vi "PULSE_OXIMETER.vi"() -> ()   [LabVIEW 2013]
uses:
  <vilib>/Instr/_visa.llb/VISA Configure Serial Port (Instr).vi
panel:
  out "Inicial Time":u32
  out "Valor Medio":string
  out "SpO2":string
  in  "A":dbl=110.0 format="%#_13g"
  in  "B":dbl=25.0 format="%#_13g"
  out "Light Intensity RED 2":i64(slide) scale=0.0..100.0
  in  "Light Intensity RED":i16(slide) scale=0.0..100.0
  out "RED":i32(graph)
  out "Light Intensity IR 2":i64(slide) scale=0.0..100.0
  out "JSON string 2":string
  out "error out":errorcluster
  out "IR":i32(graph)
  out "JSON string":string
  in  "Light Intensity IR":i64(slide) scale=0.0..100.0
  in  "Light Intensity Mode":bool
  out "AMB":i32
  out "IR":i32
  out "RED":i32
  in  "Read Count":u32=1000
  in  "End Write on Termination Character?":bool=TRUE
  in  "End Read on Termination Character?":bool=TRUE
  in  "Termination Character":u8=10 format="%.0x"
  in  "PUERTO":refnum<visa-resource-name>
  in  "START/STOP":bool
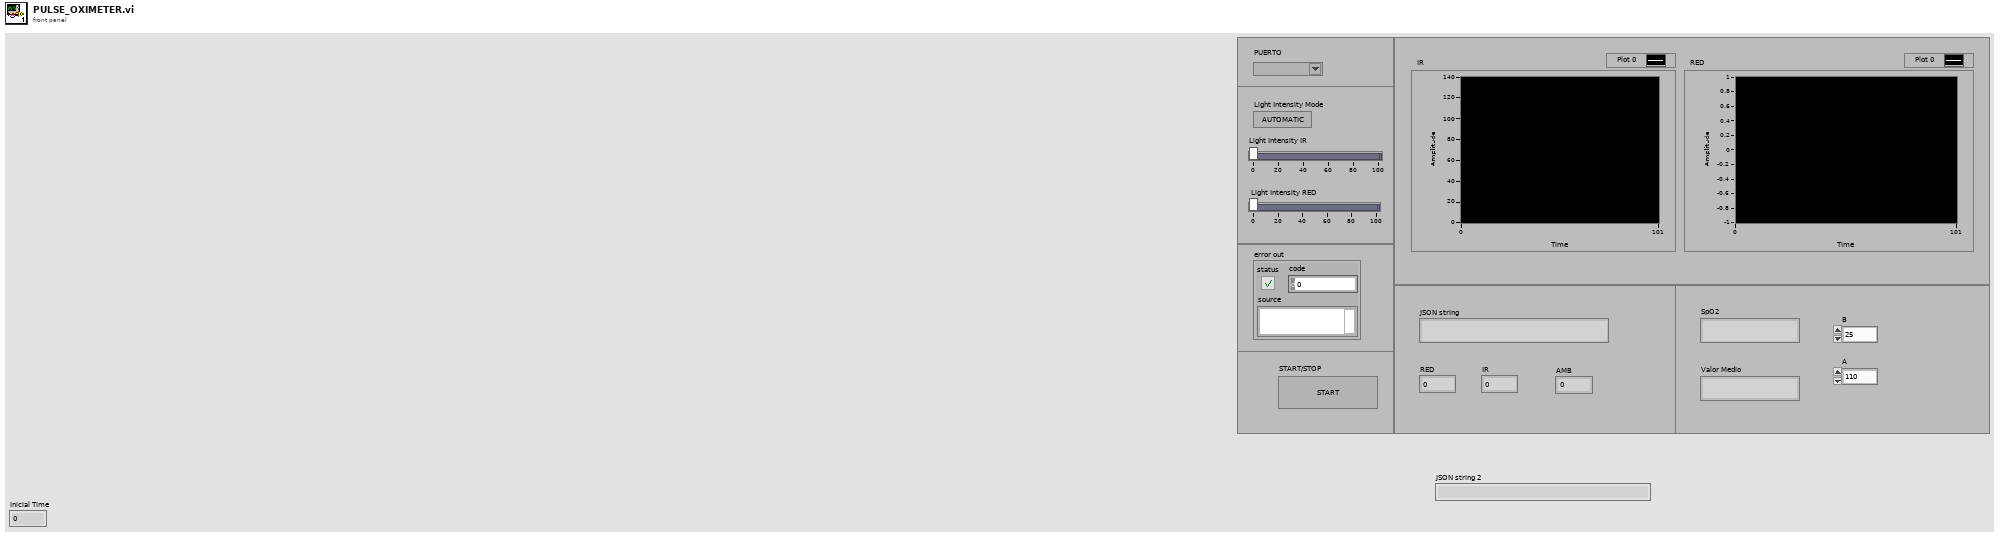
[diagram p1: front panel]
types:
  T1 = cluster{"mode":bool, "LightIntensity_IR":dbl, "status":bool, "LightIntensity_RED":dbl}
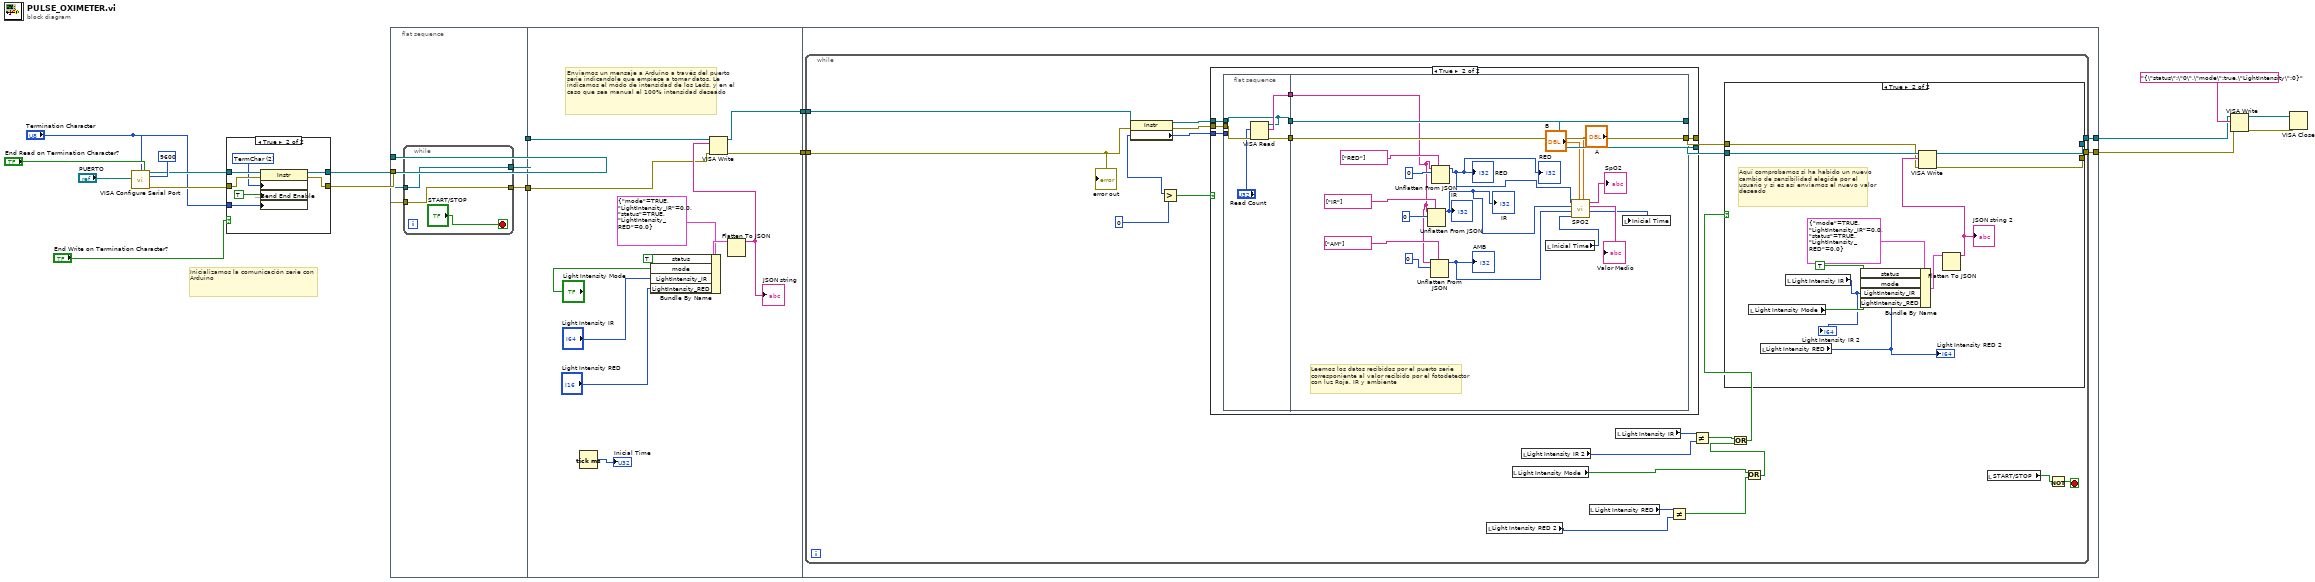
[diagram p0: block diagram]
diagram:
  # "Inicializamos la comunicación serie con Arduino"
  n1 = call-poly "VISA Configure Serial Port"("VISA resource name"="PUERTO", "termination char\n(0xA = '\\n' = LF)"="Termination Character", "Enable Termination\nChar (T)"="End Read on Termination Character?", "baud rate (9600)"=u32 9600) -> ("VISA resource name out"=w13:refnum<visa-resource-name>, "error out"=w12:errorcluster)  [unwired: 10 in]
  n2 = case shown="True" "End Write on Termination Character?" {
    tunnel: w13 -> [w19 w27]
    tunnel: w12 -> [w20 w26]
    tunnel: [w19 w25] -> w15
    tunnel: [w20 w24] -> w14
    tunnel: "Termination Character" -> [_ w22]
    frame False {
    }
    frame True {
      w23 = u16 2 items=["None", "LastBit", "TermChar", "Break"] ("Serial Settings:Serial End Mode for Writes")
      n3 = property class="Instr"(reference=w27, error in=w26, "Serial Settings:End Mode for Writes"=w23, "Message Based Settings:Send End Enable"=TRUE, "Message Based Settings:Termination Character"=w22) -> (reference out=w25:refnum<visa-resource-name>, error out=w24:errorcluster)
    }
  }
  n4 = flat-sequence {
    tunnel: w15 -> [w31]
    tunnel: w14 -> [w30]
    tunnel: [w29] -> w6
    tunnel: [w28] -> w4
    tunnel: w6 -> [w41]
    tunnel: [w40] -> w5
    tunnel: w4 -> [w39]
    tunnel: [w38] -> w3
    tunnel: w5 -> [w50]
    tunnel: w3 -> [w49]
    tunnel: [w48] -> w2
    tunnel: [w47] -> w1
    frame #0 {
      n5 = while {
        tunnel: [w34] -> w29
        tunnel: w31 -> [w34]
        tunnel: [w33] -> w28
        tunnel: w30 -> [w33]
        stop <- "START/STOP" stop-if-true
      }
    }
    frame #1 {
      # "Enviamos un mensaje a Arduino a través del puerto serie indicandole que empiece a tomar datos. Le indicamos el módo de intensidad de los Leds, y en el caso que sea manual el 100% intensidad deseado"
      n6 = Tick Count (ms)() -> (millisecond timer value=→"Inicial Time":u32)
      n7 = Bundle By Name(cluster=T1 {"mode"=TRUE, "LightIntensity_IR"=0.0, "status"=TRUE, "LightIntensity_RED"=0.0} ("input cluster"), "status"=TRUE, "mode"="Light Intensity Mode", "LightIntensity_IR"="Light Intensity IR", "LightIntensity_RED"="Light Intensity RED") -> (w46:T1)
      n8 = Flatten To JSON(anything=w46) -> (JSON string=w44:string)  [unwired: 2 in, 1 out]
      "JSON string" <- w44
      n9 = VISA Write(VISA resource name=w41, write buffer=w44, error in (no error)=w39) -> (VISA resource name out=w40:refnum<visa-resource-name>, error out=w38:errorcluster)  [unwired: 1 out]
    }
    frame #2 {
      n10 = while {
        tunnel: w50 -> [w68]
        tunnel: w49 -> [w67]
        tunnel: [w65] -> w48
        tunnel: [w64] -> w47
        stop <- w70 stop-if-true
        n11 = property class="Instr"(reference=w68, error in=w67) -> (reference out=w69:refnum<visa-resource-name>, error out=w72:errorcluster, "Serial Settings:Number of Bytes at Serial Port"=w59:u32)
        n12 = Greater?(x=w59, y=u32 0) -> (0:w60:bool)
        n13 = case shown="True" w60 {
          tunnel: w72 -> [w73 w79]
          tunnel: w59 -> [_ w78]
          tunnel: w69 -> [w74 w77]
          tunnel: [w74 w76] -> w66
          tunnel: [w73 w75] -> w63
          frame False {
          }
          frame True {
            n14 = flat-sequence {
              tunnel: w79 -> [w87]
              tunnel: w78 -> [_]
              tunnel: w77 -> [w84]
              tunnel: [w86] -> w82
              tunnel: [w85] -> w81
              tunnel: [w84] -> w80
              tunnel: [w105] -> w75
              tunnel: w82 -> [w97]
              tunnel: w81 -> [w105]
              tunnel: [w104] -> w76
              tunnel: w80 -> [w104]
              frame #0 {
                n15 = VISA Read(VISA resource name=w84, byte count="Read Count", error in (no error)=w87) -> (read buffer=w86:string, error out=w85:errorcluster)  [unwired: 2 out]
              }
              frame #1 {
                # "Leemos los datos recibidos por el puerto serie corresponiente al valor recibido por el fotodetector con luz Roja, IR y ambiente"
                n16 = Unflatten From JSON(path=string[] ["IR"] ("path 2"), JSON string=w97, type and defaults=0) -> (value=w95:i32)  [unwired: 4 in, 1 out]
                "IR" <- w95
                "IR" <- w95
                n17 = Unflatten From JSON(path=string[] ["AM"] ("path 2"), JSON string=w97, type and defaults=0) -> (value=w94:i32)  [unwired: 4 in, 1 out]
                "AMB" <- w94
                n18 = Unflatten From JSON(path=string[] ["RED"] ("path 2"), JSON string=w97, type and defaults=0) -> (value=w96:i32)  [unwired: 4 in, 1 out]
                "RED" <- w96
                "RED" <- w96
                n19 = local read "Inicial Time"() -> (w89:u32)
                n20 = call "SPO2.vi"("A"="A", "B"="B", "Inicial"=w89, "AMB"=w94, "IR"=w95, "RED"=w96) -> ("Inicial Time Out"=w88:u32, "Valor Medio"=→"Valor Medio":string, "SpO2"=→"SpO2":string)  [unwired: 3 in]
                n21 = local write "Inicial Time"(w88) -> ()
              }
            }
          }
        }
        n22 = local read "Light Intensity RED 2"() -> (w55:i64)
        n23 = local read "Light Intensity Mode"() -> (w52:bool)
        n24 = local read "Light Intensity IR 2"() -> (w61:i64)
        n25 = local read "Light Intensity RED"() -> (w56:i16)
        n26 = local read "Light Intensity IR"() -> (w62:i64)
        n27 = Not Equal?(x=w56, y=w55) -> (x != y?=w54:bool)
        n28 = Not Equal?(x=w62, y=w61) -> (x != y?=w57:bool)
        n29 = Or(x=w52, y=w54) -> (x .or. y?=w51:bool)
        n30 = Or(x=w57, y=w51) -> (x .or. y?=w53:bool)
        n31 = case shown="True" w53 {
          tunnel: w66 -> [w106 w116]
          tunnel: [w106 w115] -> w65
          tunnel: [w107 w114] -> w64
          tunnel: w63 -> [w107 w113]
          frame False {
          }
          frame True {
            # "Aquí comprobamos si ha habido un nuevo cambio de sensibilidad elegida por el usuario y si es así enviamos el nuevo valor deseado"
            n32 = local read "Light Intensity Mode"() -> (w112:bool)
            n33 = local read "Light Intensity RED"() -> (w108:i16)
            "Light Intensity RED 2" <- w108
            n34 = local read "Light Intensity IR"() -> (w111:i64)
            "Light Intensity IR 2" <- w111
            n35 = Bundle By Name(cluster=T1 {"mode"=TRUE, "LightIntensity_IR"=0.0, "status"=TRUE, "LightIntensity_RED"=0.0} ("input cluster"), "status"=TRUE, "mode"=w112, "LightIntensity_IR"=w111, "LightIntensity_RED"=w108) -> (w118:T1)
            n36 = Flatten To JSON(anything=w118) -> (JSON string=w117:string)  [unwired: 2 in, 1 out]
            "JSON string 2" <- w117
            n37 = VISA Write(VISA resource name=w116, write buffer=w117, error in (no error)=w113) -> (VISA resource name out=w115:refnum<visa-resource-name>, error out=w114:errorcluster)  [unwired: 1 out]
          }
        }
        n38 = local read "START/STOP"() -> (w71:bool)
        n39 = Not(x=w71) -> (.not. x?=w70:bool)
        "error out" <- w67
      }
    }
  }
  n40 = VISA Write(VISA resource name=w2, write buffer="{\"status\":\"0\",\"mode\":true,\"LightIntensity\":0}", error in (no error)=w1) -> (VISA resource name out=w9:refnum<visa-resource-name>, error out=w8:errorcluster)  [unwired: 1 out]
  n41 = VISA Close(VISA resource name=w9, error in (no error)=w8) -> ()  [unwired: 1 out]
